vi "Main UI.vi"(11 "FormulaLV App in":refnum<class "FormulaG App.lvclass">) -> ()   [LabVIEW 2020, in "FormulaG.lvlib" / "FormulaG App.lvclass"]
uses:
  FormulaG App.lvclass
  FormulaG-Common/Camera.ctl
  <vilib>/sklein/WebView2/Webview2 Control/WebView2 Control.xctl
  UI State.ctl
  FormulaG App.lvclass/FormulaG App.ctl
  FormulaG-Common/UI Options.ctl
  State Update.ctl
  FormulaG-Common/Car State.ctl
  FormulaG-Common/Ranges.ctl
  FormulaG-Common/Car Info.ctl
  FormulaG-Common/Car Control.ctl
  FormulaG-Common/FormulaG-Common.lvlib
  FormulaG API/FormulaG API.lvclass
  <vilib>/IlluminatedG/IG GodotServer/GodotLV/GodotServer/GodotServer.lvclass
  Pause Cmd/Pause Cmd.lvclass
  Select Cam Cmd/Select Cam Cmd.lvclass
  UI Options Cmd/UI Options Cmd.lvclass
  Reset Cmd/Reset Cmd.lvclass
panel:
  out "UI Cover":string="\n\n\n\n\n\n\n\n\n\n\n\n\n\n\n\n\nWaiting for connection to game engine..."
  out "Lap":u8
  out "Update Rate":dbl format="%.2f"
  out "Connect":dbl format="%.2f"
  out "Web":string(xcontrol)
  out "Throttle":sgl(slide) scale=0.0..1.0
  out "Speed":sgl(knob) scale=0.0..10.0
  in  "Clear Map":bool
  out "Last Lap":dbl format="%<%M:%S%3u>t"
  out "Current Lap":dbl format="%<%M:%S%3u>t"
  out "XY Graph":cluster{dbl[], dbl[]}[](graph)
  in  "Pause":bool
  out "Chart":dbl[][](graph)
  in  "Camera":T1
  in  "Reset":bool
  out "Steering":sgl(knob) scale=-1.0..1.0
  out "Connected":bool
  in  "Show Range Lines":bool
  # "Map"
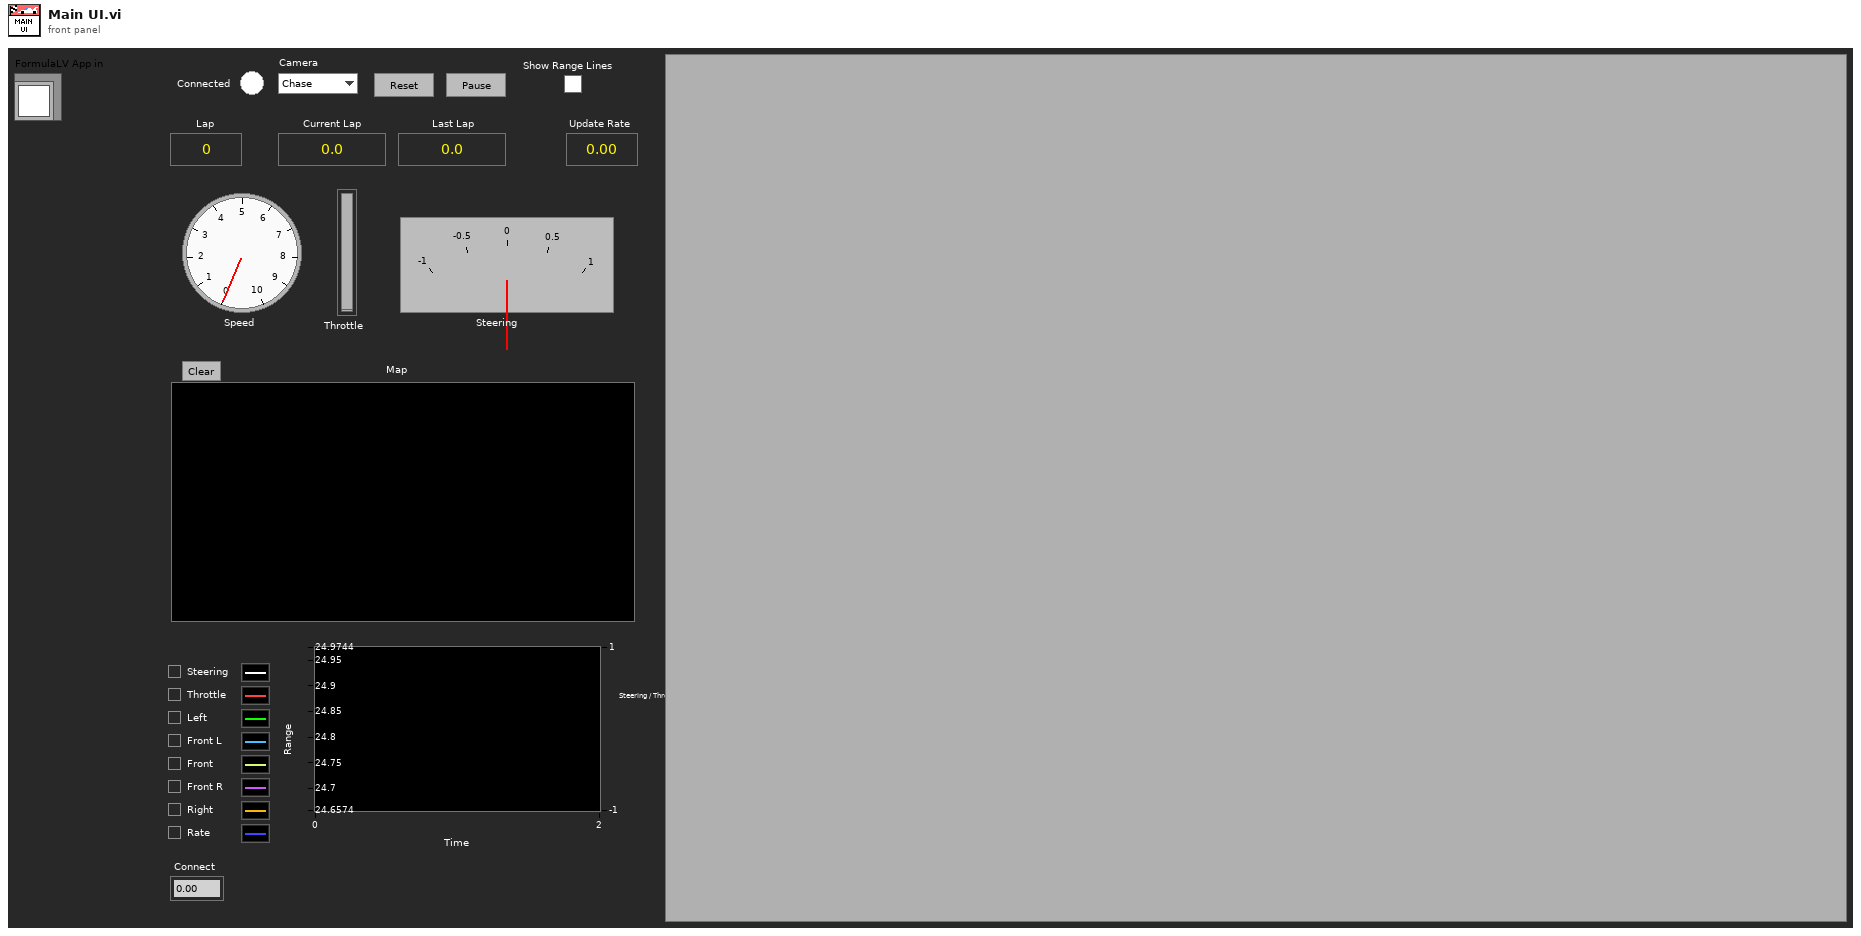
[diagram p1: front panel]
types:
  T1 = typedef "FormulaG-Common.lvlib/Camera.ctl" = enum16{"Chase", "Overhead"}
  T2 = typedef "FormulaG.lvlib/FormulaG App.lvclass/UI State.ctl" = enum16{"Init", "Connect", "Run", "Close"}
  T3 = typedef "FormulaG-Common.lvlib/UI Options.ctl" = cluster{"Range Visible":bool}
  T4 = typedef "LVRectTypeDef.ctl" = cluster{"Left":i16, "Top":i16, "Right":i16, "Bottom":i16}
  T5 = typedef "FormulaG-Common.lvlib/Car Control.ctl" = cluster{"Steering (-1 to 1)":sgl, "Throttle (0 to 1)":sgl}
  T6 = typedef "FormulaG-Common.lvlib/Car State.ctl" = cluster{"Ranges":T7, "Car Info":T8, "Current Lap":dbl, "Last Lap":dbl, "Lap":u8}
  T7 = typedef "FormulaG-Common.lvlib/Ranges.ctl" = cluster{"Front":sgl[], "Rear":sgl[]}
  T8 = typedef "FormulaG-Common.lvlib/Car Info.ctl" = cluster{"Speed":sgl, "X":sgl, "Y":sgl, "Heading":sgl}
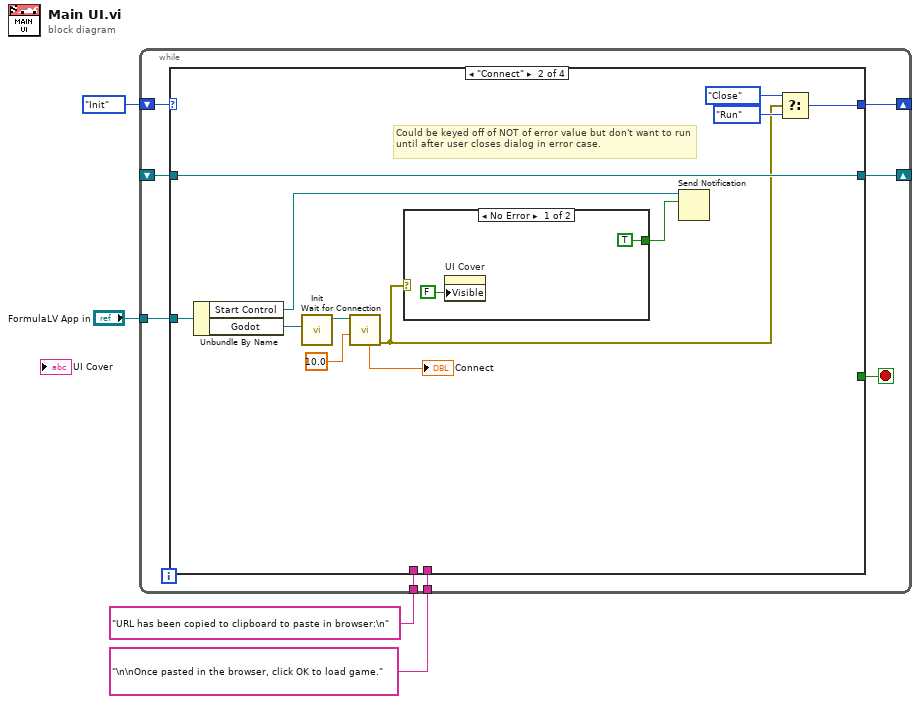
[diagram p0: block diagram]
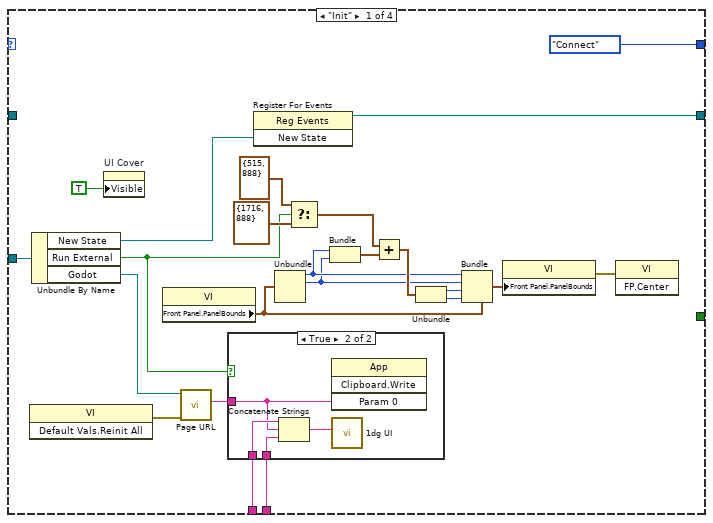
[diagram p2: hidden frame]
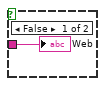
[diagram p3: hidden frame]
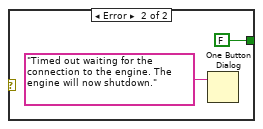
[diagram p4: hidden frame]
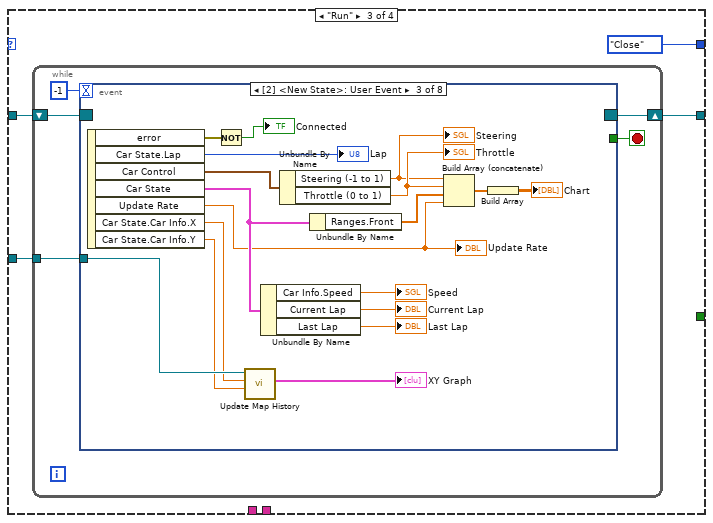
[diagram p5: hidden frame]
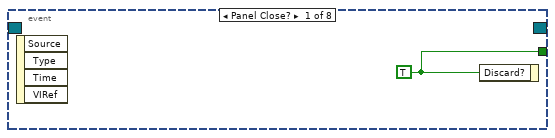
[diagram p6: hidden frame]
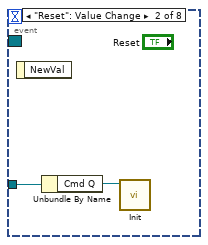
[diagram p7: hidden frame]
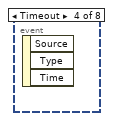
[diagram p8: hidden frame]
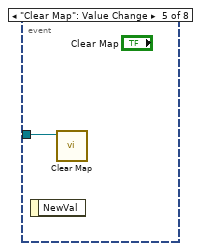
[diagram p9: hidden frame]
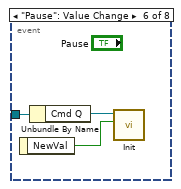
[diagram p10: hidden frame]
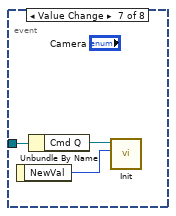
[diagram p11: hidden frame]
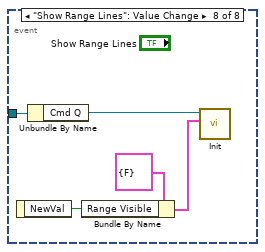
[diagram p12: hidden frame]
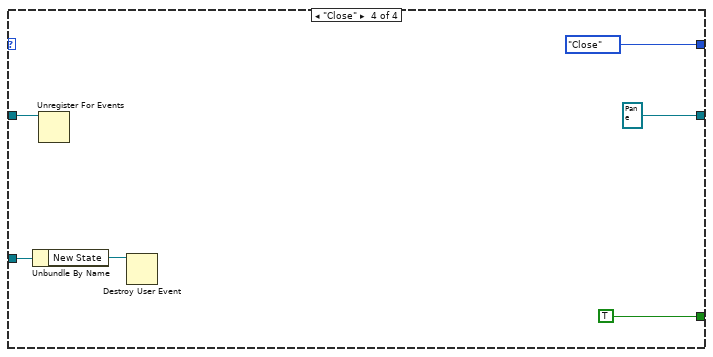
[diagram p13: hidden frame]
diagram:
  n1 = while {
    tunnel: "FormulaLV App in" -> [w12]
    shift-right: [w9] -> _
    shift-left: UI_State."Init" ("UI State") -> [w11]
    shift-right: [w8] -> _
    shift-left: _ -> [w7]
    tunnel: "URL has been copied to clipboard to paste in browser:\n" -> [w6]
    tunnel: "\n\nOnce pasted in the browser, click OK to load game." -> [w5]
    stop <- w10 stop-if-true
    n2 = case shown="\"Connect\"" w11 {
      tunnel: w12 -> [w32 w49 w60 w100]
      tunnel: [_ _ _ TRUE] -> w10
      tunnel: [UI_State."Connect" ("UI State") w52 UI_State."Close" ("UI State") UI_State."Close" ("UI State")] -> w9
      tunnel: [w28 w45 w57 refnum<event-registration> refnum ("Event Registration Refnum")] -> w8
      tunnel: w7 -> [_ w45 w58 w101]
      tunnel: w6 -> [w15 _ _ _]
      tunnel: w5 -> [w14 _ _ _]
      frame "Init" {
        n3 = invoke class="VI" method="Default Vals.Reinit All"() -> (error out=w35:errorcluster)  [unwired: 3 in, 2 out]
        n4 = Unbundle By Name(w32) -> ("New State"=w29:refnum<user-event>, "Run External"=w25:bool, "Godot"=w33:refnum<class "GodotServer.lvclass">)
        n5 = property on="UI Cover" class="Str"("Visible"=TRUE) -> ()  [unwired: 2 in, 2 out]
        n6 = property class="VI"() -> ("Front Panel.PanelBounds"=w23:T4)  [unwired: 2 in, 2 out]
        n7 = call <vilib>:"Page URL.vi"("error in (no error)"=w35, "GodotServer in"=w33) -> ("Page URL"=w34:string)  [unwired: 7 in, 2 out]
        n8 = case shown="True" w25 {
          tunnel: w34 -> [w36 w38]
          tunnel: w15 -> [_ w40]
          tunnel: w14 -> [_ w39]
          frame False {
            "Web" <- w36
          }
          frame True {
            n9 = Concatenate Strings(w40, w38, w39) -> (w37:string)
            n10 = invoke class="App" method="Clipboard.Write"("Param 0"=w38) -> ()  [unwired: 3 in, 4 out]
            n11 = call "1dg UI.vi"("String"=w37) -> ()  [unwired: 11 in]
          }
        }
        n12 = register-events(w29) -> (reference out=w28:refnum<event-registration>)  [unwired: 2 in, 1 out]
        n13 = Unbundle(w23) -> ("Left"=w17:i16, "Top"=w16:i16)  [unwired: 2 out]
        n14 = Select(t=cluster{i16, i16} {515, 888} ("External"), s=w25, f=cluster{i16, i16} {1716, 888} ("External")) -> (s? t:f=w21:cluster{i16, i16})
        n15 = Bundle("Left"=w17, "Top"=w16) -> (w24:cluster{"Left":i16, "Top":i16})  [unwired: 1 in]
        n16 = Add(x=w21, y=w24) -> (x+y=w20:cluster{i16, i16})
        n17 = Unbundle(w20) -> (w18:i16, w19:i16)
        n18 = Bundle(cluster=w23, "Left"=w17, "Top"=w16, "Right"=w18, "Bottom"=w19) -> (w22:T4)
        n19 = property class="VI"("Front Panel.PanelBounds"=w22) -> (error out=w13:errorcluster)  [unwired: 2 in, 1 out]
        n20 = invoke class="VI" method="FP.Center"(error in=w13) -> ()  [unwired: 2 in, 3 out]
      }
      frame "Connect" {
        # "Could be keyed off of NOT of error value but don't want to run until after user closes dialog in error case."
        n21 = Unbundle By Name(w49) -> ("Start Control"=w43:refnum<notifier>, "Godot"=w48:refnum<class "GodotServer.lvclass">)
        n22 = call "Init.vi"("Godot"=w48) -> ("FormulaG API out"=w47:refnum<class "FormulaG API.lvclass">)  [unwired: 9 in, 1 out]
        n23 = call "Wait for Connection.vi"("Timeout S (30)"=10.0, "FormulaG API in"=w47) -> ("error out"=w42:errorcluster, "Time"=→"Connect":dbl)  [unwired: 7 in, 1 out]
        n24 = case shown="No Error" w42 {
          tunnel: [TRUE FALSE] -> w41
          frame No Error {
            n25 = property on="UI Cover" class="Str"("Visible"=FALSE) -> ()  [unwired: 2 in, 2 out]
          }
          frame Error {
            n26 = One Button Dialog(message="Timed out waiting for the connection to the engine. The engine will now shutdown.") -> ()  [unwired: 1 in, 1 out]
          }
        }
        n27 = Send Notification(notification=w41, notifier=w43) -> ()  [unwired: 1 in, 2 out]
        n28 = Select(t=UI_State."Close" ("UI State"), s=w42, f=UI_State."Run" ("UI State")) -> (s? t:f=w52:T2)
      }
      frame "Run" {
        n29 = while {
          tunnel: w60 -> [w64]
          shift-right: [w61] -> w57
          shift-left: w58 -> [w62]
          stop <- w65 stop-if-true
          n30 = event shown="[2] <New State>: User Event" {
            selector: w62 -> [_ _ _ _ _ _ _ _]
            dyn-events: [_ _ _ _ _ _ _ _] -> w61
            timeout: -1 -> [_ _ _ _ _ _ _ _]
            tunnel: [w66 _ _ _ _ _ _ _] -> w65
            tunnel: w64 -> [_ w68 w83 _ w87 w90 w93 w98]
            event Panel Close? {
              w66 = TRUE ("Discard?")
              n31 = event-data() -> ()  [unwired: 1 in, 4 out]
              n32 = event-data("Discard?"=w66) -> ()  [unwired: 1 in, 1 out]
            }
            event "Reset": Value Change {
              n33 = event-data() -> ()  [unwired: 1 in, 1 out]
              n34 = Unbundle By Name(w68) -> ("Cmd Q"=w67:refnum<queue>)
              n35 = call "Init.vi"("Cmd Q"=w67) -> ()  [unwired: 11 in]
            }
            event User Event {
              n36 = event-data() -> ("error"=w70:errorcluster, "Car State.Lap"=→"Lap":u8, "Car Control"=w79:T5, "Car State"=w75:T6, "Update Rate"=w71:dbl, "Car State.Car Info.X"=w82:sgl, "Car State.Car Info.Y"=w81:sgl)  [unwired: 1 in]
              "Update Rate" <- w71
              n37 = Not(x=w70) -> (.not. x?=→"Connected":bool)
              n38 = call "Update Map History.vi"("Y"=w81, "X"=w82, "FormulaG App in"=w83) -> ("XY Graph"=→"XY Graph":cluster{dbl[], dbl[]}[])  [unwired: 6 in, 2 out]
              n39 = Unbundle By Name(w75) -> ("Car Info.Speed"=→"Speed":sgl, "Current Lap"=→"Current Lap":dbl, "Last Lap"=→"Last Lap":dbl)
              n40 = Unbundle By Name(w79) -> ("Steering (-1 to 1)"=w73:sgl, "Throttle (0 to 1)"=w74:sgl)
              "Steering" <- w73
              "Throttle" <- w74
              n41 = Unbundle By Name(w75) -> ("Ranges.Front"=w78:sgl[])
              n42 = Build Array (concatenate)(w73, w74, w78, w71) -> (w77:dbl[])
              n43 = Build Array(w77) -> (→"Chart":dbl[][])
            }
            event Timeout {
              n44 = event-data() -> ()  [unwired: 1 in, 3 out]
            }
            event "Clear Map": Value Change {
              n45 = event-data() -> ()  [unwired: 1 in, 1 out]
              n46 = call "Clear Map.vi"("FormulaG App in"=w87) -> ()  [unwired: 9 in, 2 out]
            }
            event "Pause": Value Change {
              n47 = event-data() -> ("NewVal"=w89:bool)  [unwired: 1 in]
              n48 = Unbundle By Name(w90) -> ("Cmd Q"=w88:refnum<queue>)
              n49 = call "Init.vi"("Pause"=w89, "Cmd Q"=w88) -> ()  [unwired: 9 in, 1 out]
            }
            event Value Change {
              n50 = event-data() -> ("NewVal"=w92:T1)  [unwired: 1 in]
              n51 = Unbundle By Name(w93) -> ("Cmd Q"=w91:refnum<queue>)
              n52 = call "Init.vi"("Camera"=w92, "Cmd Q"=w91) -> ()  [unwired: 9 in, 1 out]
            }
            event "Show Range Lines": Value Change {
              n53 = event-data() -> ("NewVal"=w96:bool)  [unwired: 1 in]
              n54 = Unbundle By Name(w98) -> ("Cmd Q"=w95:refnum<queue>)
              n55 = Bundle By Name(cluster=T3 {"Range Visible"=FALSE} ("UI Options"), "Range Visible"=w96) -> (w94:T3)
              n56 = call "Init.vi"("UI Options"=w94, "Cmd Q"=w95) -> ()  [unwired: 9 in, 1 out]
            }
          }
        }
      }
      frame "Close" {
        n57 = Unbundle By Name(w100) -> ("New State"=w99:refnum<user-event>)
        n58 = Unregister For Events(event registration refnum=w101) -> ()  [unwired: 1 in, 1 out]
        n59 = Destroy User Event(user event=w99) -> ()  [unwired: 1 in, 1 out]
      }
    }
  }
